vi "Window Orign Caller Zero Zero.vi"(11 "error in (no error)":errorcluster) -> (15 "error out":errorcluster)   [LabVIEW 2018]
uses:
  <vilib>/Utility/miscctls.llb/LVPointTypeDef.ctl
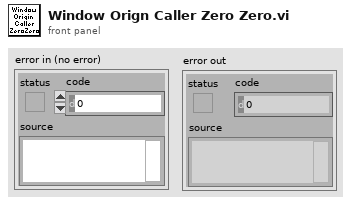
[diagram p1: front panel]
types:
  T1 = typedef "LVPointTypeDef.ctl" = cluster{"Horizontal":i16, "Vertical":i16}
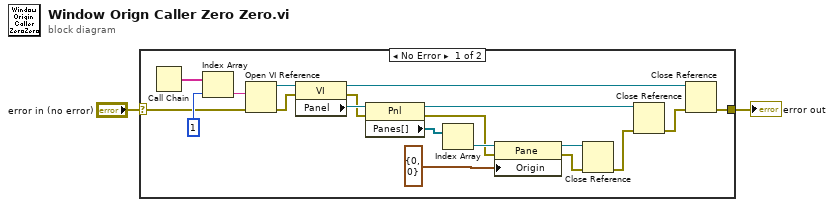
[diagram p0: block diagram]
diagram:
  n1 = case shown="No Error" "error in (no error)" {
    selector: "error in (no error)" -> [w3 w22]
    tunnel: [w4 w22] -> w2
    frame No Error {
      n2 = Call Chain() -> (call chain=w21:string[])
      n3 = Index Array(array=w21, index=1) -> (element=w19:string)
      n4 = Open VI Reference(vi path=w19, error in (no error)=w3) -> (vi reference=w6:refnum<vi>, error out=w5:errorcluster)  [unwired: 4 in]
      n5 = property class="VI"(reference=w6, error in=w5) -> (reference out=w15:refnum<vi>, error out=w14:errorcluster, "Panel"=w18:refnum<vi>)
      n6 = property class="Pnl"(reference=w18, error in=w14) -> (reference out=w10:refnum<vi>, error out=w13:errorcluster, "Panes[]"=w17:refnum<vi>[])
      n7 = Index Array(array=w17) -> (element=w16:refnum<vi>)  [unwired: 1 in]
      n8 = property class="Pane"(reference=w16, error in=w13, "Origin"=T1 {"Horizontal"=0, "Vertical"=0}) -> (reference out=w12:refnum<vi>, error out=w11:errorcluster)
      n9 = Close Reference(reference=w12, error in (no error)=w11) -> (error out=w9:errorcluster)
      n10 = Close Reference(reference=w10, error in (no error)=w9) -> (error out=w8:errorcluster)
      n11 = Close Reference(reference=w15, error in (no error)=w8) -> (error out=w4:errorcluster)
    }
    frame Error {
    }
  }
  "error out" <- w2
